vi "Set Signal Configuration.vi"(8 "error in (no error)":errorcluster, 10 "Configuration":T1, 11 "IO Class in":refnum<class "Signal.lvclass">) -> (0 "error out":errorcluster, 3 "IO Class out":refnum<class "Signal.lvclass">)   [LabVIEW 2015, in "Signal.lvclass"]
uses:
  Signal.lvclass
  Configuration.ctl
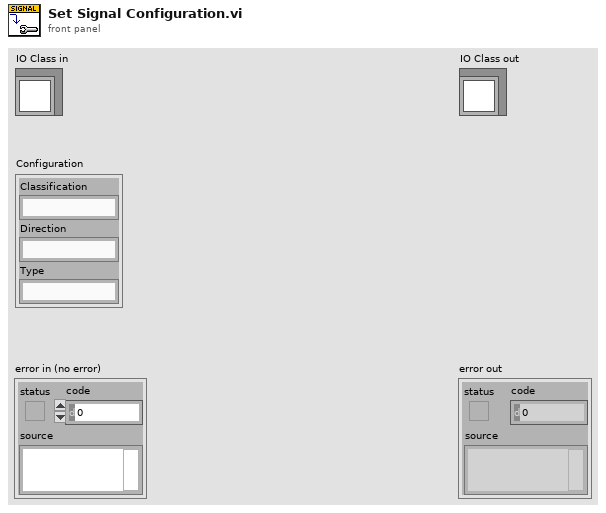
[diagram p1: front panel]
types:
  T1 = typedef "Signal.lvclass/Configuration.ctl" = cluster{"Classification":string, "Direction":string, "Type":string}
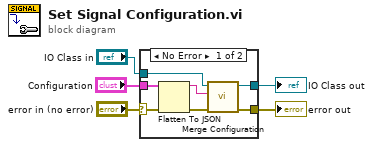
[diagram p0: block diagram]
diagram:
  n1 = case shown="No Error" "error in (no error)" {
    selector: "error in (no error)" -> [w10 w14]
    tunnel: [w6 w14] -> w4
    tunnel: [w9 w13] -> w2
    tunnel: "IO Class in" -> [w12 w13]
    tunnel: "Configuration" -> [w11 _]
    frame No Error {
      n2 = Flatten To JSON(anything=w11, error in (no error)=w10) -> (JSON string=w8:string, 11:w7:errorcluster)  [unwired: 1 in]
      n3 = call "Merge Configuration.vi"("error in (no error)"=w7, "Additional Configuration"=w8, "IO Class in"=w12) -> ("error out"=w6:errorcluster, "IO Class out"=w9:refnum<class "Signal.lvclass">)  [unwired: 7 in]
    }
    frame Error {
    }
  }
  "error out" <- w4
  "IO Class out" <- w2
